vi "Lab03_LabViewFileReadWrite_Bennett.vi"() -> ()   [LabVIEW 2017]
uses:
  <vilib>/Analysis/baseanly.llb/Mean (DBL).vi
  <vilib>/Utility/file.llb/Read Delimited Spreadsheet (DBL).vi
  <vilib>/Utility/file.llb/Write Delimited Spreadsheet (DBL).vi
  <vilib>/Analysis/NI_AALBase.lvlib
panel:
  out "Max Value":dbl
  out "Min Value":dbl
  out "Manipulated":waveform(dbl)(graph)
  out "Num Pts":dbl
  out "Mean":dbl
  out "Data Read":dbl[](array[numeric])
  out "Original":waveform(dbl)(graph)
  # "ELEC3800: IoT                                               Lab03                                          Matt Bennett\nFall 2017                                                                                                               09/15/17"
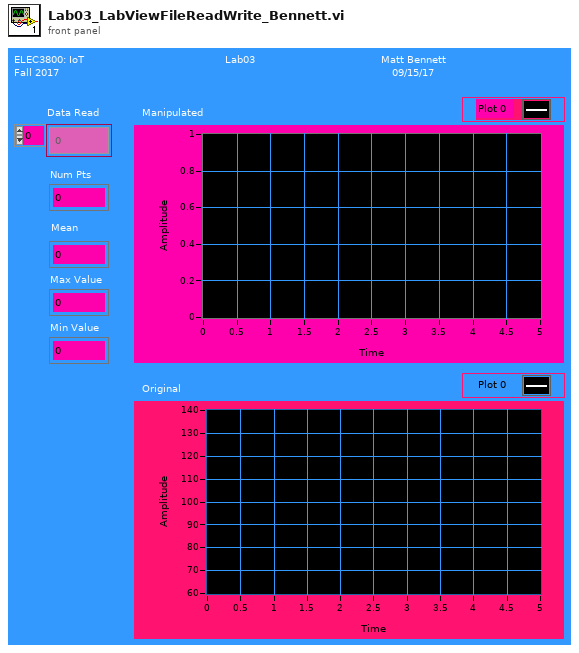
[diagram p1: front panel]
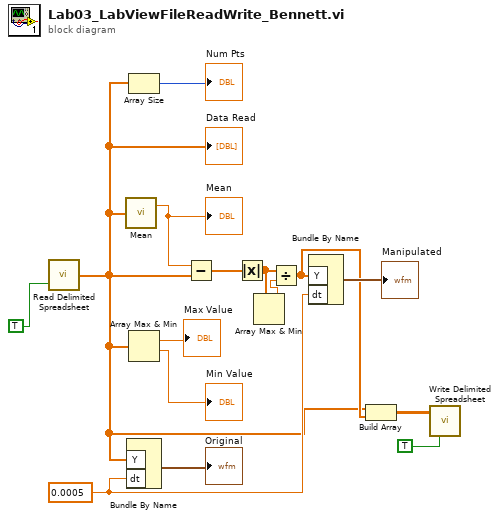
[diagram p0: block diagram]
diagram:
  w9 = 0.0005
  n1 = call-poly <vilib>:"Read Delimited Spreadsheet.vi"("transpose? (F)"=TRUE) -> ("first row"=w5:dbl[])  [unwired: 9 in, 5 out]
  "Data Read" <- w5
  n2 = call-poly <vilib>:"Mean.vi"("X"=w5) -> ("mean"=w11:dbl)  [unwired: 1 out]
  "Mean" <- w11
  n3 = Bundle By Name("Y"=w5, "dt"=w9) -> (→"Original":waveform(dbl))  [unwired: 1 in]
  n4 = Array Size(array=w5) -> (size(s)=→"Num Pts":i32)
  n5 = Array Max & Min(array=w5) -> (max value=→"Max Value":dbl, min value=→"Min Value":dbl)  [unwired: 2 out]
  n6 = Subtract(x=w11, y=w5) -> (x-y=w10:dbl[])
  n7 = Absolute Value(x=w10) -> (abs(x)=w2:dbl[])
  n8 = Array Max & Min(array=w2) -> (max value=w1:dbl)  [unwired: 3 out]
  n9 = Divide(x=w2, y=w1) -> (x/y=w6:dbl[])
  n10 = Bundle By Name("Y"=w6, "dt"=w9) -> (→"Manipulated":waveform(dbl))  [unwired: 1 in]
  n11 = Build Array(w5, w6) -> (w4:dbl[][])
  n12 = call-poly <vilib>:"Write Delimited Spreadsheet.vi"("2D data"=w4, "transpose? (no:F)"=TRUE) -> ()  [unwired: 12 in, 2 out]
